vi "MapOwnWindow.vi"() -> ()   [LabVIEW 2014]
uses:
  <vilib>/Utility/miscctls.llb/LVCursorListTypeDef.ctl
  <vilib>/Platform/TimedLoop/XDataNode/timing_clust.ctl
  <vilib>/Platform/TimedLoop/XDataNode/nitl_modes.ctl
  <vilib>/Platform/TimedLoop/XDataNode/wakeup.ctl
  <vilib>/Platform/TimedLoop/XDataNode/XDataNode.xnode
  <vilib>/Platform/TimedLoop/XDataNode/XDNodeRunTimeDep.lvlib
panel:
  in  "Cursor List":T1
  in  "Eta_ship":dbl[](array[numeric])=[0.0, 0.0, 0.0]
  in  "Close":bool
  out "East":dbl
  out "North":dbl
  in  "Update View":bool
  in  "Trace Buffer":i32=50
  in  "Range":dbl=30.0
  in  "Auto Center ROV":bool
  in  "Eta":dbl[](array[numeric])=[0.0, 3.0, 0.0, 0.0, 0.0, 0.0]
  in  "Eta_des":dbl[](array[numeric])
  in  "Eta_est":dbl[](array[numeric])=[0.0, 0.0, 0.0, 0.0, 0.0, 0.0]
  out "XY Graph":cluster{dbl[], dbl[]}[](graph)
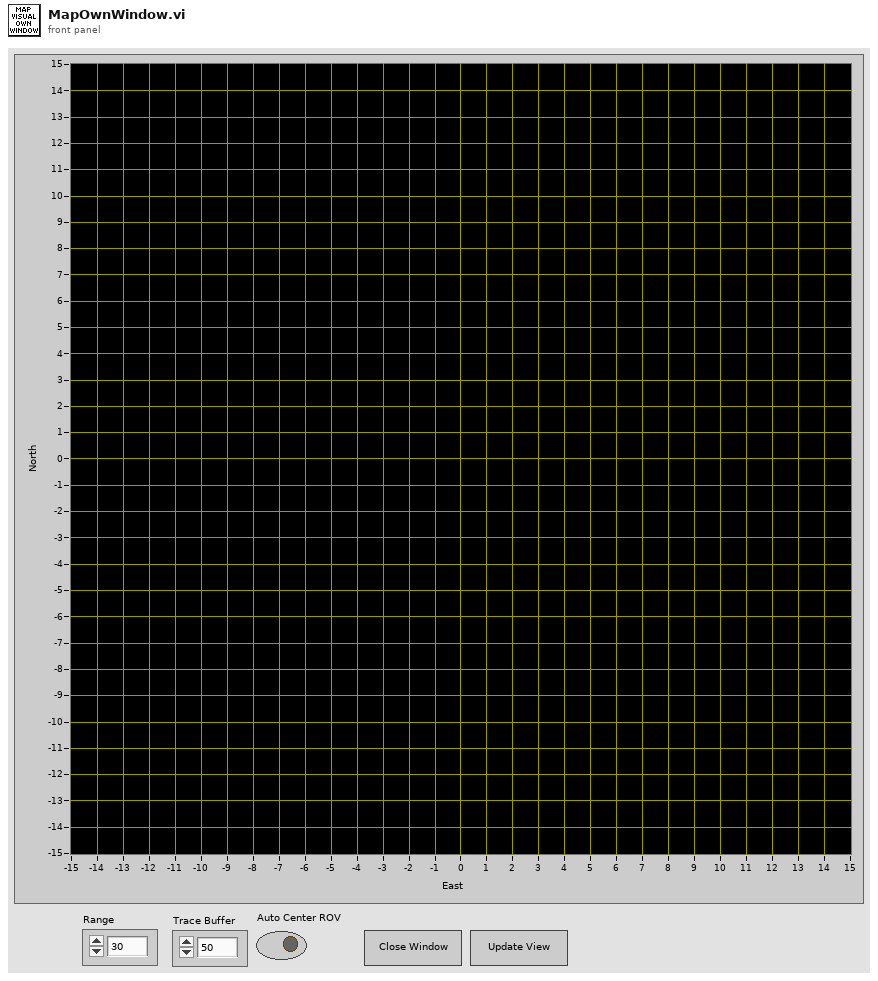
[diagram p1: front panel]
types:
  T1 = typedef "LVCursorListTypeDef.ctl" = cluster{"Name":string, "Color":u32, "Style":u8, "Point Style":u8, "Name Visible":bool, "Allow Drag":bool, "Cursor Mode":u32, "Plot":i32, "Index":i32, "Position":cluster{"X":dbl, "Y":dbl}, "X Scale":u32, "Y Scale":u32, "Watch Plots":i32[], "Watch All Plots":bool, "Plot Area":i32, "Label Offset":cluster{"X":dbl, "Y":dbl}}[]
  T2 = typedef "XDNodeRunTimeDep.lvlib/timing_clust.ctl" = cluster{"Expected End [f-1]":u64, "Actual End [f-1]":u64, "Finished Late? [f-1]":bool, "Expected End [i-1]":u64, "Actual End [i-1]":u64, "Finished Late? [i-1]":bool, "Expected Start [i]":u64, "Actual Start [i]":u64, "Expected Start [f]":u64, "Actual Start [f]":u64, "Source Name":string, "Structure Name":string, "Period":i64, "Deadline":i64, "Offset":i64, "Start":i64, "Priority":i32, "Timeout":i32, "Mode":T3, "Wakeup Reason":T4, "Error":errorcluster, "Source Type":string, "Secondary Source Type":string, "Global End Time":u64, "Global Start Time":u64, "Frame Duration":u64, "Iteration Duration":u64, "Assigned CPU":i32, "I/O Scan Engine Mode":u32}
  T3 = typedef "XDNodeRunTimeDep.lvlib/nitl_modes.ctl" = enum32{"No Change", "Process missed periods, maintain original phase", "Discard missed periods, maintain original phase", "Process missed periods, ignore original phase", "Discard missed periods, ignore original phase"}
  T4 = typedef "XDNodeRunTimeDep.lvlib/wakeup.ctl" = enum32{"Normal", "Aborted", "Asynchronous wakeup", "Timing source error", "Timed loop error", "Timeout"}
  T5 = typedef "LVRangeTypeDef.ctl" = cluster{"Minimum":dbl, "Maximum":dbl, "Increment":dbl, "Minor Increment":dbl, "Start":dbl}
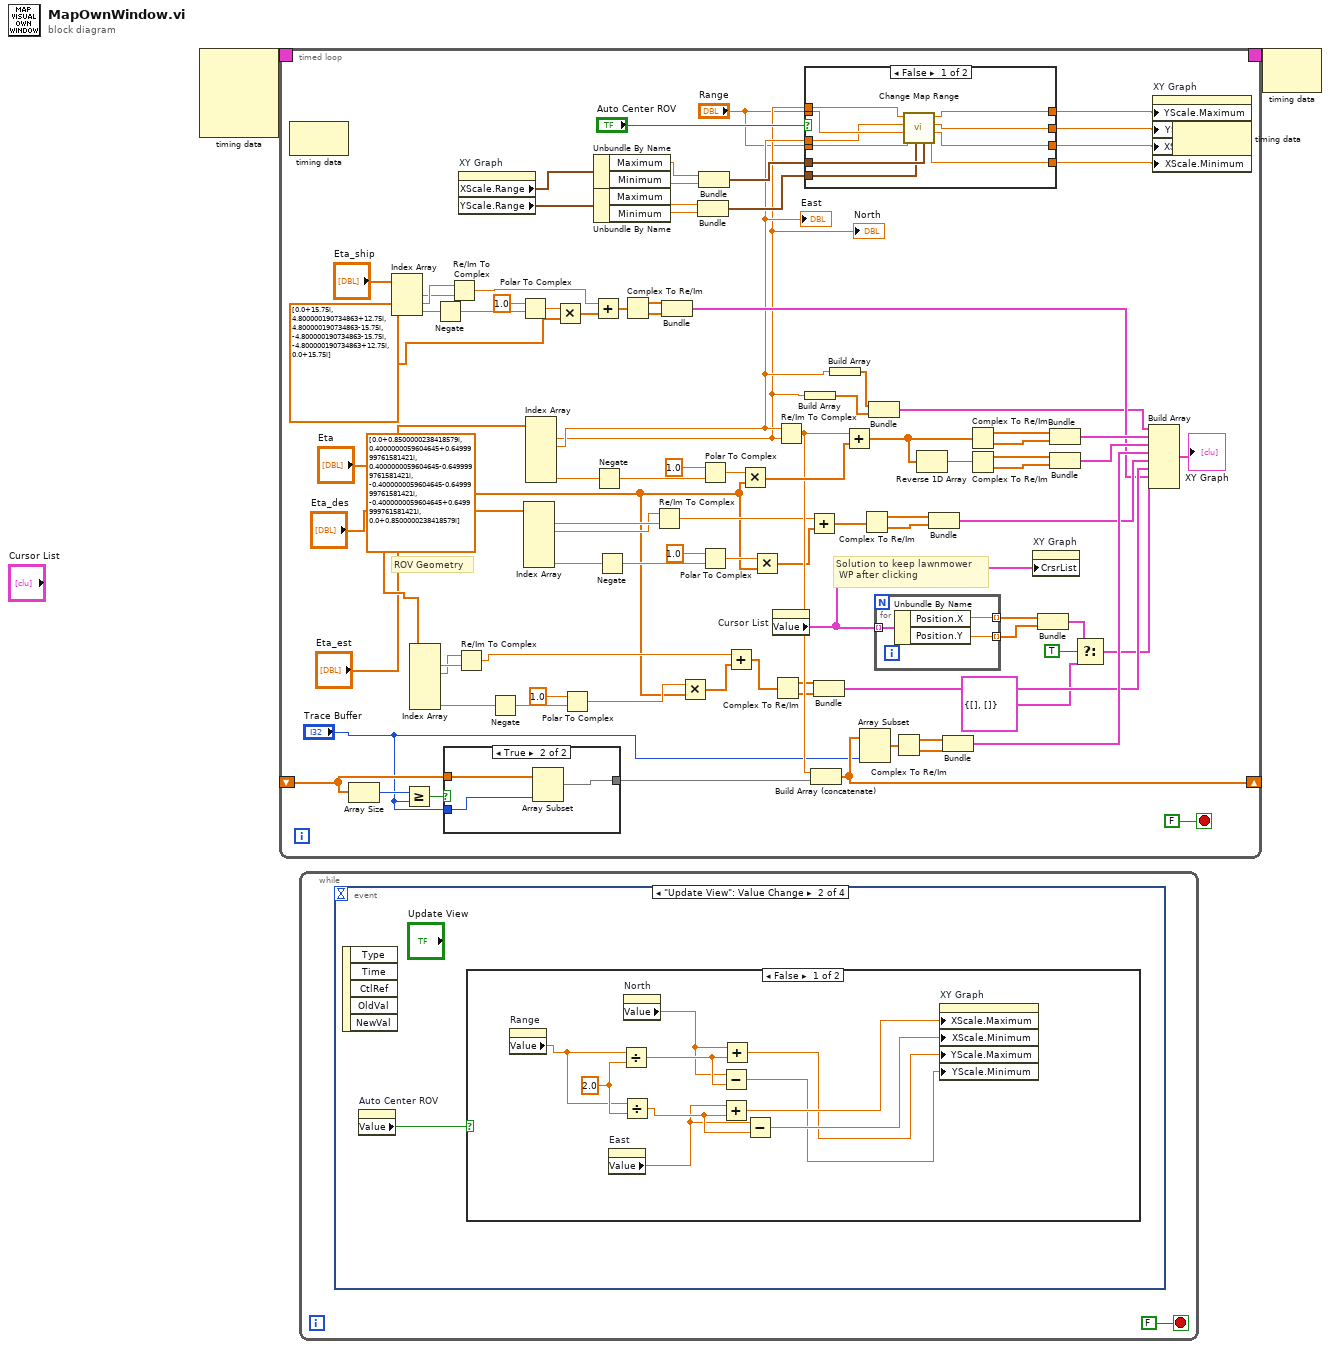
[diagram p0: block diagram]
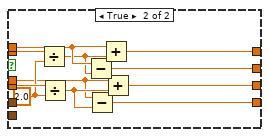
[diagram p2: hidden frame]
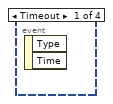
[diagram p4: hidden frame]
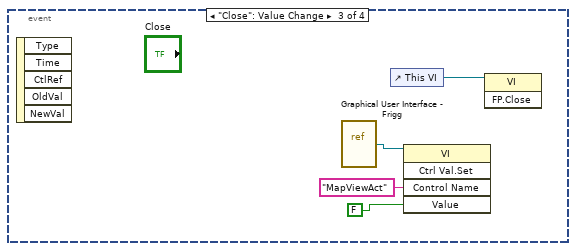
[diagram p6: hidden frame]
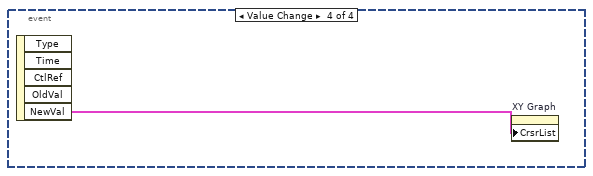
[diagram p7: hidden frame]
diagram:
  n1 = node-c288() -> (w2:T2)  [unwired: 4 in]
  n2 = timed-loop {
    shift-right: [w79] -> _
    shift-left: _ -> [w82]
    timing: w2 -> [_]
    timing-out: [_] -> w1
    stop <- FALSE stop-if-true
    w30 = csg[] [0.0+0.85i, 0.4+0.65i, 0.4-0.65i, -0.4-0.65i, -0.4+0.65i, 0.0+0.85i] ("XYi")
    # "Solution to keep lawnmower\n WP after clicking"
    # "ROV Geometry"
    n3 = node-c288() -> ()  [unwired: 1 in, 1 out]
    n4 = Array Size(array=w82) -> (size(s)=w83:i32)
    n5 = Index Array(array="Eta_ship") -> (element #1=w31:dbl, element #2=w32:dbl, element #3=w28:dbl)  [unwired: 3 in]
    n6 = Greater Or Equal?(x=w83, y="Trace Buffer") -> (x >= y?=w84:bool)
    n7 = Index Array(array="Eta") -> (element #1=w54:dbl, element #2=w53:dbl, element #6=w52:dbl)  [unwired: 6 in, 3 out]
    n8 = Negate(x=w28) -> (-x=w27:dbl)
    n9 = case shown="True" w84 {
      tunnel: "Trace Buffer" -> [_ w126]
      tunnel: w82 -> [w123 w125]
      tunnel: [w123 w124] -> w80
      frame False {
      }
      frame True {
        n10 = Array Subset(array=w125, length=w126) -> (w124:cdb[])  [unwired: 1 in]
      }
    }
    n11 = Re/Im To Complex(1:w31, 2:w32) -> (0:w24:cdb)
    n12 = Re/Im To Complex(1:w54, 2:w53) -> (0:w47:cdb)
    n13 = property on="XY Graph" class="XYGraph (strict)"() -> ("XScale.Range"=w43:T5, "YScale.Range"=w42:T5)  [unwired: 2 in, 2 out]
    n14 = Negate(x=w52) -> (-x=w51:dbl)
    n15 = Polar To Complex(1:w27, 2:1.0) -> (0:w26:cdb)
    n16 = Index Array(array="Eta_des") -> (element #1=w63:dbl, element #2=w62:dbl, element #6=w66:dbl)  [unwired: 6 in, 3 out]
    n17 = Index Array(array="Eta_est") -> (element #1=w17:dbl, element #2=w19:dbl, element #6=w96:dbl)  [unwired: 6 in, 3 out]
    "North" <- w17
    "East" <- w19
    n18 = Multiply(x=w26, y=csg[] [0.0+15.75i, 4.8+12.75i, 4.8-15.75i, -4.8-15.75i, -4.8+12.75i, 0.0+15.75i] ("XYi")) -> (x*y=w25:cdb[])
    n19 = Polar To Complex(1:w51, 2:1.0 ("r")) -> (0:w49:cdb)
    n20 = Add(x=w24, y=w25) -> (x+y=w23:cdb[])
    n21 = Unbundle By Name(w43) -> ("Maximum"=w73:dbl, "Minimum"=w72:dbl)
    n22 = Unbundle By Name(w42) -> ("Maximum"=w71:dbl, "Minimum"=w70:dbl)
    n23 = Negate(x=w96) -> (-x=w95:dbl)
    n24 = Negate(x=w66) -> (-x=w64:dbl)
    n25 = Complex To Re/Im(x + iy=w23) -> (x=w21:dbl[], y=w22:dbl[])
    n26 = Re/Im To Complex(1:w63, 2:w62) -> (0:w60:cdb)
    n27 = Bundle(w21, w22) -> (w20:cluster{dbl[], dbl[]})  [unwired: 1 in]
    n28 = Multiply(x=w49, y=w30) -> (x*y=w48:cdb[])
    n29 = Bundle("Maximum"=w71, "Minimum"=w70) -> (w68:cluster{"Maximum":dbl, "Minimum":dbl})  [unwired: 1 in]
    n30 = Bundle("Maximum"=w73, "Minimum"=w72) -> (w69:cluster{"Maximum":dbl, "Minimum":dbl})  [unwired: 1 in]
    n31 = Polar To Complex(1:w95, 2:1.0) -> (0:w93:cdb)
    n32 = Polar To Complex(1:w64, 2:1.0) -> (0:w61:cdb)
    n33 = Add(x=w47, y=w48) -> (x+y=w45:cdb[])
    n34 = Multiply(x=w93, y=w30) -> (x*y=w92:cdb[])
    n35 = Multiply(x=w61, y=w30) -> (x*y=w59:cdb[])
    n36 = property on="Cursor List" class="Arr (strict)"() -> ("Value"=w8:T1)  [unwired: 2 in, 2 out]
    n37 = Complex To Re/Im(x + iy=w45) -> (x=w44:dbl[], y=w46:dbl[])
    n38 = Re/Im To Complex(1:w17, 2:w19) -> (0:w81:cdb)
    n39 = case shown="False" "Auto Center ROV" {
      tunnel: "Range" -> [w107 w122]
      tunnel: "Range" -> [w106 w121]
      tunnel: w17 -> [w104 w119]
      tunnel: w19 -> [w105 w116]
      tunnel: [w111 w115] -> w41
      tunnel: [w110 w114] -> w40
      tunnel: [w109 w113] -> w39
      tunnel: [w108 w112] -> w38
      tunnel: w69 -> [w103 _]
      tunnel: w68 -> [w102 _]
      frame False {
        n40 = call "Change Map Range.vi"("Current East Bounds"=w103, "Current North Bounds"=w102, "Range East"=w106, "Range North"=w107, "East"=w105, "North"=w104) -> ("East Min"=w108:dbl, "East Max"=w109:dbl, "North Min"=w110:dbl, "North Max"=w111:dbl)  [unwired: 2 in]
      }
      frame True {
        w120 = 2.0
        n41 = Divide(x=w122, y=w120) -> (x/y=w118:dbl)
        n42 = Divide(x=w121, y=w120) -> (x/y=w117:dbl)
        n43 = Subtract(x=w119, y=w118) -> (x-y=w114:dbl)
        n44 = Subtract(x=w116, y=w117) -> (x-y=w112:dbl)
        n45 = Add(x=w119, y=w118) -> (x+y=w115:dbl)
        n46 = Add(x=w116, y=w117) -> (x+y=w113:dbl)
      }
    }
    n47 = Build Array(w17) -> (w16:dbl[])
    n48 = Add(x=w60, y=w59) -> (x+y=w58:cdb[])
    n49 = Build Array (concatenate)(w81, w80) -> (w79:cdb[])
    n50 = Bundle(w44, w46) -> (w36:cluster{dbl[], dbl[]})  [unwired: 1 in]
    n51 = Build Array(w19) -> (w18:dbl[])
    n52 = Add(x=w81, y=w92) -> (x+y=w91:cdb[])
    n53 = Array Subset(array=w79, length="Trace Buffer") -> (w78:cdb[])  [unwired: 1 in]
    n54 = Complex To Re/Im(x + iy=w58) -> (x=w57:dbl[], y=w56:dbl[])
    n55 = Bundle(w18, w16) -> (w15:cluster{dbl[], dbl[]})  [unwired: 1 in]
    n56 = for {
      tunnel: w8 -> [w99] mode=indexing
      tunnel: [w98] -> w10 mode=indexing
      tunnel: [w97] -> w9 mode=indexing
      n57 = Unbundle By Name(w99) -> ("Position.X"=w98:dbl, "Position.Y"=w97:dbl)
    }
    n58 = Complex To Re/Im(x + iy=w78) -> (x=w77:dbl[], y=w76:dbl[])
    n59 = Reverse 1D Array(array=w91) -> (reversed array=w90:cdb[])
    n60 = Bundle(w57, w56) -> (w37:cluster{dbl[], dbl[]})  [unwired: 1 in]
    n61 = Bundle(w77, w76) -> (w55:cluster{dbl[], dbl[]})  [unwired: 1 in]
    n62 = Complex To Re/Im(x + iy=w91) -> (x=w75:dbl[], y=w89:dbl[])
    n63 = Complex To Re/Im(x + iy=w90) -> (x=w88:dbl[], y=w87:dbl[])
    n64 = property on="XY Graph" class="XYGraph (strict)"("CrsrList"=w8) -> ()  [unwired: 2 in, 2 out]
    n65 = Bundle(w10, w9) -> (w7:cluster{dbl[], dbl[]})  [unwired: 1 in]
    n66 = Bundle(w75, w89) -> (w86:cluster{dbl[], dbl[]})  [unwired: 1 in]
    n67 = Bundle(w88, w87) -> (w85:cluster{dbl[], dbl[]})  [unwired: 1 in]
    n68 = Select(t=w7, s=TRUE, f=cluster{dbl[], dbl[]} {[], []}) -> (s? t:f=w6:cluster{dbl[], dbl[]})
    n69 = Build Array(w15, w86, w85, w55, w37, w36, w20, w6) -> (→"XY Graph":cluster{dbl[], dbl[]}[])
    n70 = property on="XY Graph" class="XYGraph (strict)"("YScale.Maximum"=w41, "YScale.Minimum"=w40, "XScale.Maximum"=w39, "XScale.Minimum"=w38) -> ()  [unwired: 2 in, 2 out]
    n71 = node-c288() -> ()  [unwired: 1 in, 1 out]
  }
  n72 = while {
    stop <- FALSE stop-if-true
    n73 = event shown="[1] \"Update View\": Value Change" {
      selector: _ -> [_ _ _ _]
      dyn-events: _ -> [_ _ _ _]
      timeout: _ -> [_ _ _ _]
      event Timeout {
        n74 = event-data() -> ()  [unwired: 1 in, 2 out]
      }
      event "Update View": Value Change {
        n75 = event-data() -> ()  [unwired: 1 in, 5 out]
        n76 = property on="Auto Center ROV" class="Bool (strict)"() -> ("Value"=w128:bool)  [unwired: 2 in, 2 out]
        n77 = case shown="False" w128 {
          frame False {
            w138 = 2.0
            n78 = property on="Range" class="DigNum (strict)"() -> ("Value"=w129:dbl)  [unwired: 2 in, 2 out]
            n79 = property on="East" class="DigNum (strict)"() -> ("Value"=w130:dbl)  [unwired: 2 in, 2 out]
            n80 = Divide(x=w129, y=w138) -> (x/y=w137:dbl)
            n81 = Divide(x=w129, y=w138) -> (x/y=w136:dbl)
            n82 = property on="North" class="DigNum (strict)"() -> ("Value"=w131:dbl)  [unwired: 2 in, 2 out]
            n83 = Subtract(x=w131, y=w137) -> (x-y=w132:dbl)
            n84 = Add(x=w130, y=w136) -> (x+y=w135:dbl)
            n85 = Add(x=w131, y=w137) -> (x+y=w133:dbl)
            n86 = Subtract(x=w130, y=w136) -> (x-y=w134:dbl)
            n87 = property on="XY Graph" class="XYGraph (strict)"("XScale.Maximum"=w135, "XScale.Minimum"=w134, "YScale.Maximum"=w133, "YScale.Minimum"=w132) -> ()  [unwired: 2 in, 2 out]
          }
          frame True {
          }
        }
      }
      event "Close": Value Change {
        n88 = event-data() -> ()  [unwired: 1 in, 5 out]
        n89 = vi-ref "Graphical User Interface - Frigg.vi"() -> (w141:refnum<vi>)
        n90 = control-ref of="This VI"() -> (w142:refnum<vi>)
        n91 = invoke class="VI" method="Ctrl Val.Set"(reference=w141, "Control Name"="MapViewAct", "Value"=FALSE) -> ()  [unwired: 2 in, 5 out]
        n92 = invoke class="VI" method="FP.Close"(reference=w142) -> ()  [unwired: 2 in, 3 out]
      }
      event Value Change {
        n93 = event-data() -> ("NewVal"=w143:T1)  [unwired: 1 in, 4 out]
        n94 = property on="XY Graph" class="XYGraph (strict)"("CrsrList"=w143) -> ()  [unwired: 2 in, 2 out]
      }
    }
  }
  n95 = node-c288(w1) -> ()  [unwired: 1 out]
